vi "VIBuildProject.vi"(8 "error in (no error)":errorcluster, 10 "Parameters":string[](array[string])) -> (0 "error out":errorcluster)   [LabVIEW 2013]
uses:
  VIProject/VIProject.lvlib
panel:
  out "Current Spec":string
  out "Current Target":string
  out "Total":i32
  out "Progress":i32(slide) scale=0.0..1.0
  # "Path to project"
  # "Target name"
  # "Spec name"
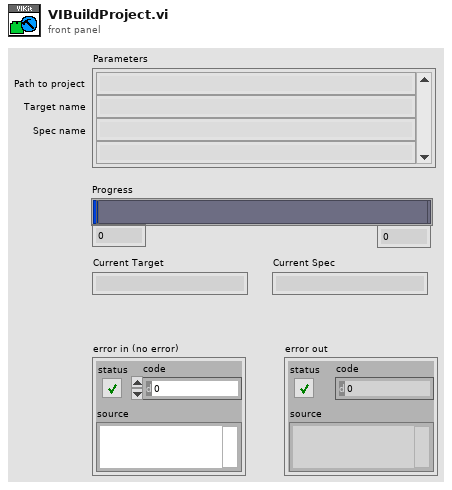
[diagram p1: front panel]
types:
  T1 = typedef "VIProject.lvlib/VPTargetBuildSpecs.ctl" = cluster{"Target Name":string, "Build Specifications":T2[]}
  T2 = typedef "VIProject.lvlib/VPBuildSpecInformation.ctl" = cluster{"Name":string, "Type":string}
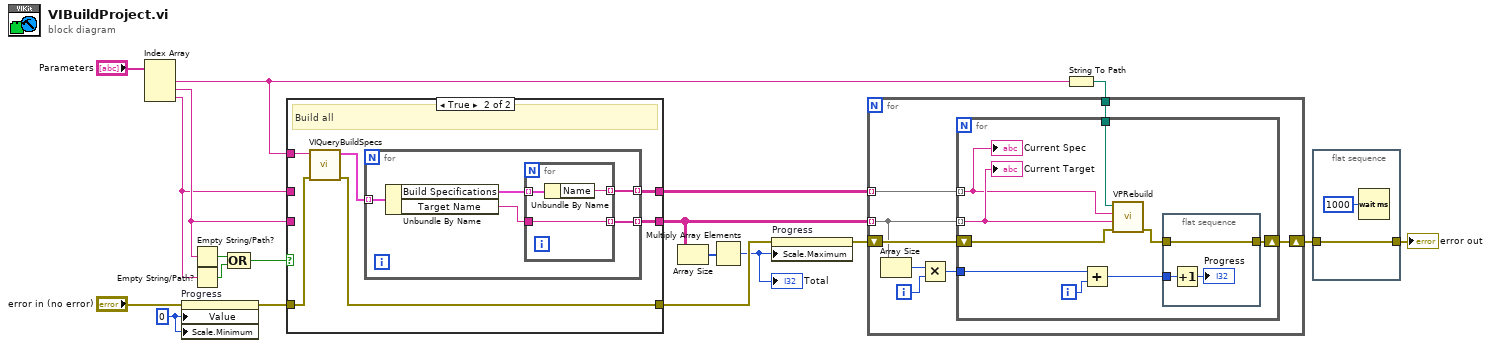
[diagram p0: block diagram]
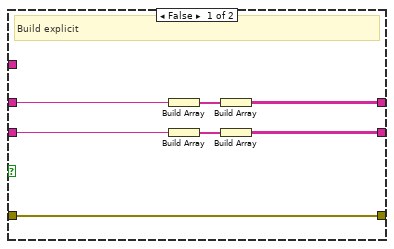
[diagram p2: hidden frame]
diagram:
  w7 = 0 ("Progress")
  n1 = Index Array(array="Parameters") -> (element #1=w15:string, element #2=w14:string, element #3=w13:string)  [unwired: 3 in]
  n2 = property on="Progress" class="Slide (strict)"(error in="error in (no error)", "Value"=w7, "Scale.Minimum"=w7) -> (error out=w10:errorcluster)  [unwired: 1 in, 1 out]
  n3 = Empty String/Path?(string/path=w14) -> (empty?=w18:bool)
  n4 = Empty String/Path?(string/path=w13) -> (empty?=w17:bool)
  n5 = Compound Arithmetic op=OR(w18, w17) -> (w16:bool)
  n6 = case shown="True" w16 {
    tunnel: w15 -> [_ w32]
    tunnel: [w24 w27] -> w9
    tunnel: w13 -> [w26 _]
    tunnel: w14 -> [w22 _]
    tunnel: w10 -> [w21 w30]
    tunnel: [w21 w29] -> w6
    tunnel: [w20 w28] -> w4
    frame False {
      # "Build explicit"
      n7 = Build Array(w26) -> (w25:string[])
      n8 = Build Array(w22) -> (w23:string[])
      n9 = Build Array(w25) -> (w24:string[][])
      n10 = Build Array(w23) -> (w20:string[][])
    }
    frame True {
      # "Build all"
      n11 = call "VIQueryBuildSpecs.vi"("Error In"=w30, "Project Path"=w32) -> ("Error Out"=w29:errorcluster, "Targets"=w31:T1[])  [unwired: 8 in]
      n12 = for {
        tunnel: w31 -> [w37] mode=indexing
        tunnel: [w35] -> w27 mode=indexing
        tunnel: [w33] -> w28 mode=indexing
        n13 = Unbundle By Name(w37) -> ("Build Specifications"=w36:T2[], "Target Name"=w34:string)
        n14 = for {
          tunnel: w36 -> [w40] mode=indexing
          tunnel: [w39] -> w35 mode=indexing
          tunnel: w34 -> [w38]
          tunnel: [w38] -> w33 mode=indexing
          n15 = Unbundle By Name(w40) -> ("Name"=w39:string)
        }
      }
    }
  }
  n16 = Array Size(array=w4) -> (size(s)=w8:i32[])
  n17 = Multiply Array Elements(1:w8) -> (0:w3:i32)
  "Total" <- w3
  n18 = property on="Progress" class="Slide (strict)"(error in=w6, "Scale.Maximum"=w3) -> (error out=w5:errorcluster)  [unwired: 1 in, 1 out]
  n19 = String To Path(string=w15) -> (path=w12:path)
  n20 = for {
    tunnel: w9 -> [w48] mode=indexing
    tunnel: w4 -> [w44] mode=indexing
    tunnel: w12 -> [w47]
    shift-right: [w45] -> w1
    shift-left: w5 -> [w46]
    i -> [w42]
    n21 = Array Size(array=w44) -> (size(s)=w43:i32)
    n22 = Multiply(x=w43, y=w42) -> (x*y=w41:i32)
    n23 = for {
      tunnel: w48 -> [w51] mode=indexing
      tunnel: w44 -> [w52] mode=indexing
      tunnel: w47 -> [w57]
      shift-right: [w49] -> w45
      shift-left: w46 -> [w56]
      tunnel: w41 -> [w54]
      i -> [w55]
      n24 = Add(x=w54, y=w55) -> (x+y=w53:i32)
      n25 = call "VPRebuild.vi"("error in (no error)"=w56, "Name of target"=w52, "Name of build specification"=w51, "Path to project"=w57) -> ("error out"=w50:errorcluster)  [unwired: 6 in, 1 out]
      n26 = flat-sequence {
        tunnel: w53 -> [w60]
        tunnel: w50 -> [w59]
        tunnel: [w59] -> w49
        frame #0 {
          n27 = Increment(x=w60) -> (x+1=→"Progress":i32)
        }
      }
      "Current Spec" <- w51
      "Current Target" <- w52
    }
  }
  n28 = flat-sequence {
    tunnel: [w61] -> w2
    tunnel: w1 -> [w61]
    frame #0 {
      n29 = Wait (ms)(milliseconds to wait=u32 1000) -> ()  [unwired: 1 out]
    }
  }
  "error out" <- w2
